vi "All time (SILAR).vi"(0 "Необходимое кол-во циклов":i32=1, 1 "Режим погружения подложки":u16(ring) items=["Частичное", "Полное"], 2 "Подъема подложки над раствором":dbl[](array[numeric])=[2.9, 2.9, 0.0, 0.0], 3 "Подъема подложки из раствора":dbl[](array[numeric])=[1.9, 1.9, 0.0, 0.0], 4 "Нахождения в растворе (секунды)":dbl[](array[numeric])=[1.0, 1.0, 0.0, 0.0] caption="Время нахождения в растворе (секунды)", 5 "Кол-во используемых растворов":i32(ring)=1 items=["Один"=1, "Два"=2, "Три"=3, "Четыре"=4], 6 "Высота стакана (мм)":dbl=50.0, 7 "Кол-во погружений в каждый стакан за один цикл":i32[](array[numeric])=[1, 1, 0, 0], 8 "Задержка после подъема из раствора (секунды)":dbl[](array[numeric])=[1.0, 1.0, 0.0, 0.0], 9 "Опускания подложки в раствор":dbl[](array[numeric])=[1.9, 1.9, 0.0, 0.0], 11 "Глубина погружения в раствор (мм)":dbl[](array[numeric])=[7.0, 7.0, 0.0, 0.0], 12 "Опускания подложки до раствора":dbl[](array[numeric])=[2.9, 2.9, 0.0, 0.0], 13 "Высота подложки (мм)":dbl=10.0, 14 "Кол-во жидкости в каждом стакане (мм)":dbl[](array[numeric])=[25.0, 25.0, 25.0, 25.0]) -> (10 "Все время":timestamp=timestamp(-14394 s since 1904-01-01) format="%<%H:%M:%S>T", 15 "Все время":dbl=6.0)   [LabVIEW 2016]
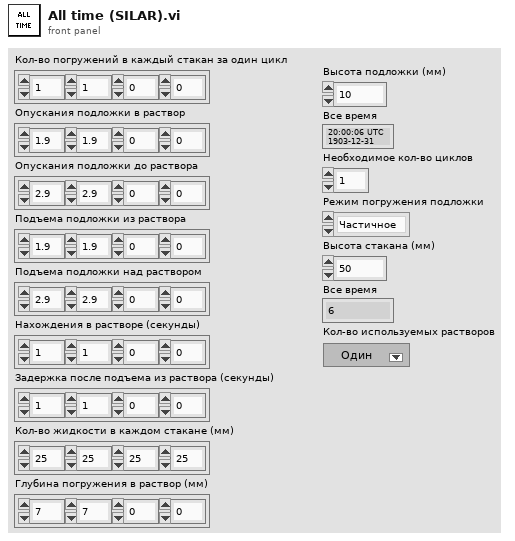
[diagram p1: front panel]
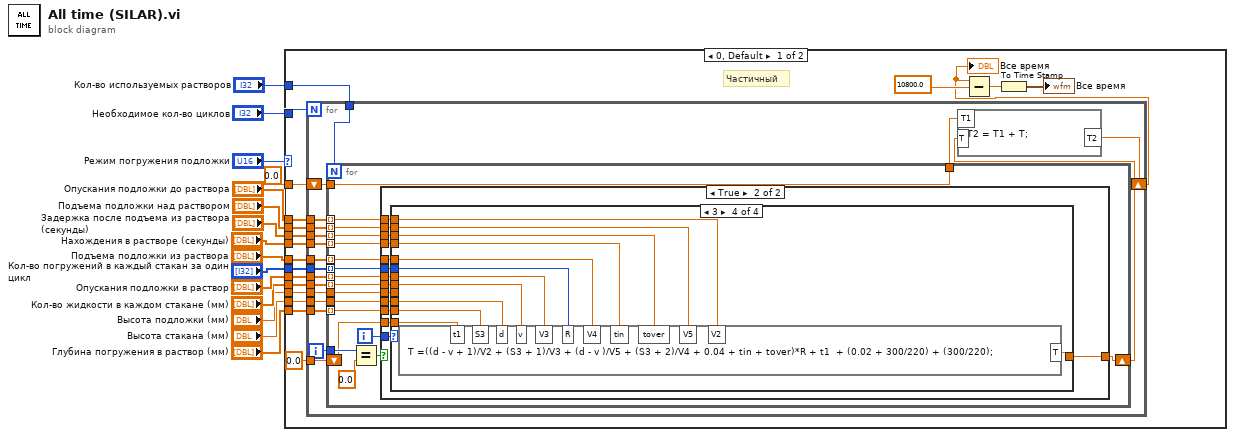
[diagram p0: block diagram]
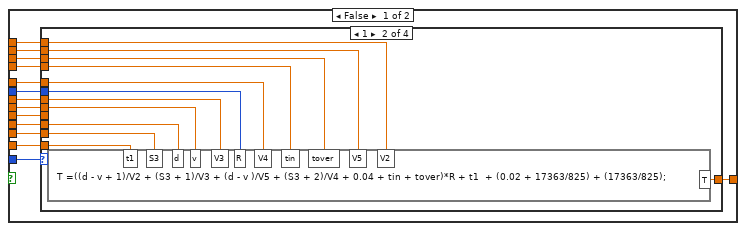
[diagram p2: hidden frame]
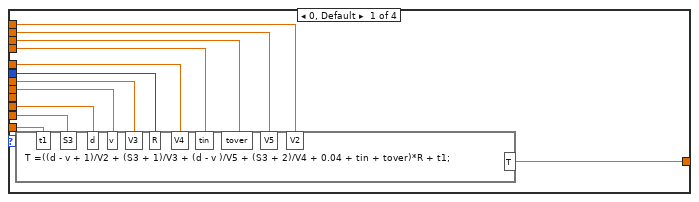
[diagram p3: hidden frame]
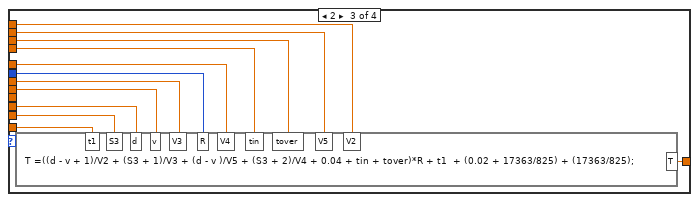
[diagram p4: hidden frame]
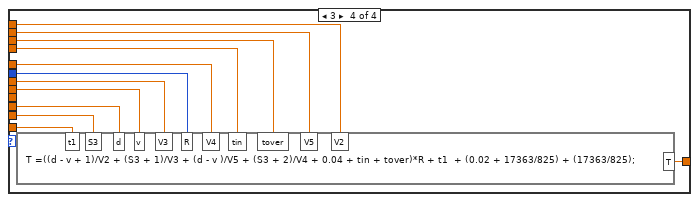
[diagram p5: hidden frame]
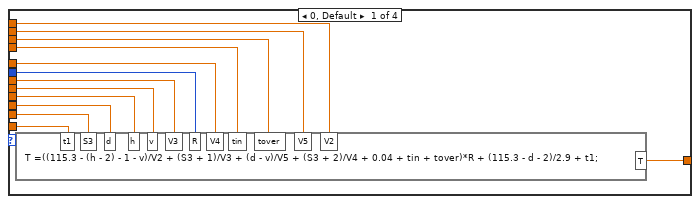
[diagram p6: hidden frame]
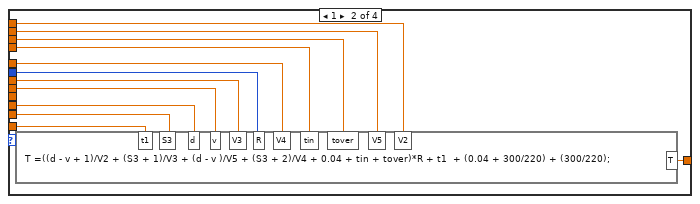
[diagram p7: hidden frame]
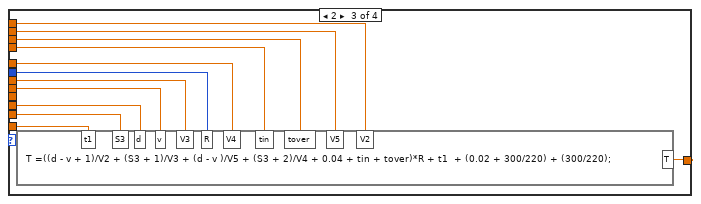
[diagram p8: hidden frame]
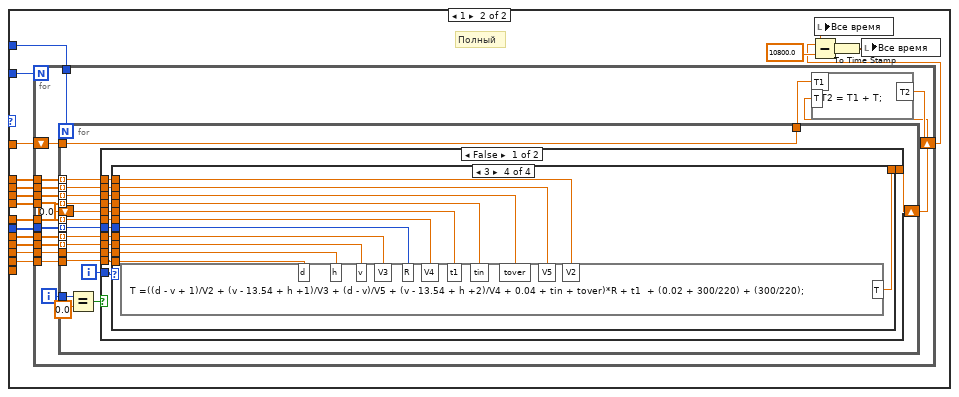
[diagram p9: hidden frame]
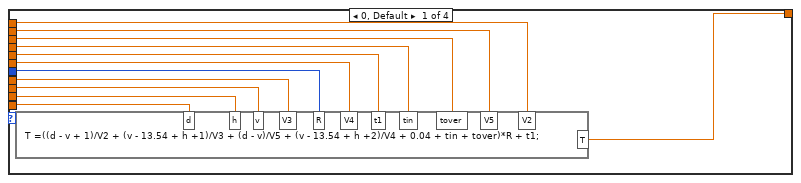
[diagram p10: hidden frame]
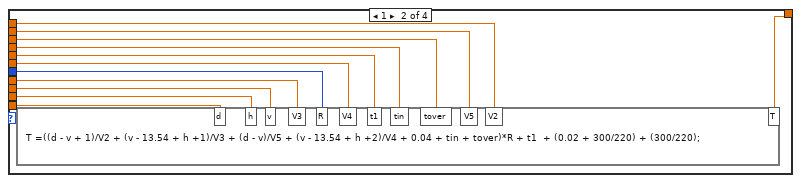
[diagram p11: hidden frame]
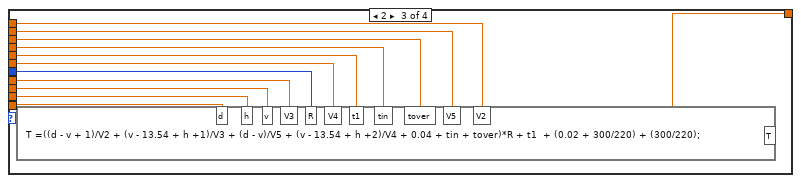
[diagram p12: hidden frame]
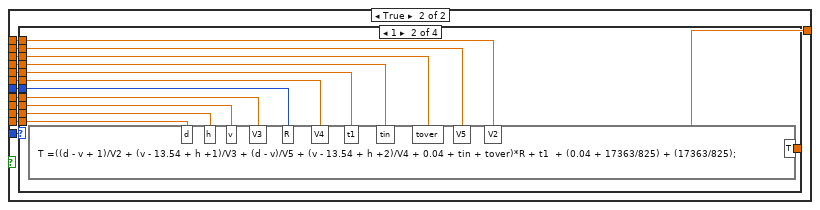
[diagram p13: hidden frame]
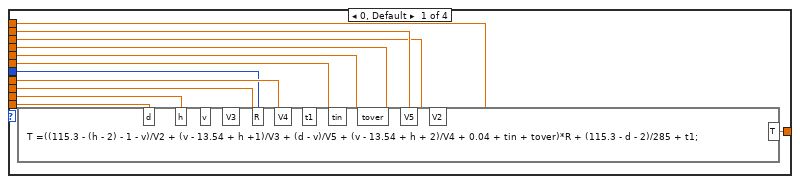
[diagram p14: hidden frame]
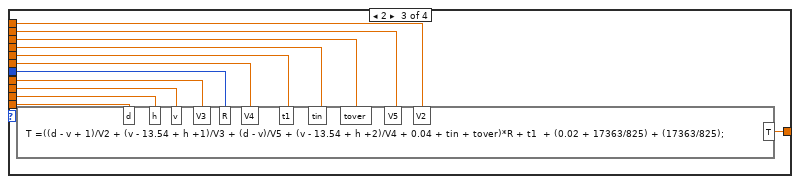
[diagram p15: hidden frame]
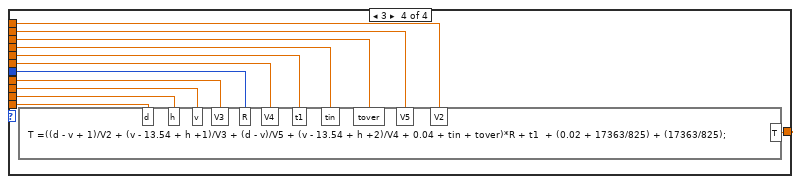
[diagram p16: hidden frame]
diagram:
  n1 = case shown="0, Default" "Режим погружения подложки" {
    tunnel: "Кол-во используемых растворов" -> [w33 w210]
    tunnel: "Задержка после подъема из раствора (секунды)" -> [w30 w206]
    tunnel: "Нахождения в растворе (секунды)" -> [w29 w205]
    tunnel: "Подъема подложки из раствора" -> [w28 w204]
    tunnel: "Кол-во погружений в каждый стакан за один цикл" -> [w22 w203]
    tunnel: "Опускания подложки в раствор" -> [w27 w202]
    tunnel: "Необходимое кол-во циклов" -> [w34 w209]
    tunnel: "Глубина погружения в раствор (мм)" -> [w26 _]
    tunnel: "Кол-во жидкости в каждом стакане (мм)" -> [w25 w201]
    tunnel: "Высота подложки (мм)" -> [w24 w200]
    tunnel: "Высота стакана (мм)" -> [w23 w199]
    tunnel: "Опускания подложки до раствора" -> [w32 w208]
    tunnel: "Подъема подложки над раствором" -> [w31 w207]
    tunnel: 0.0 -> [w18 w197]
    frame 0, Default {
      # "Частичный"
      n2 = for {
        N: w34 -> [_]
        tunnel: w33 -> [w52]
        shift-right: [w37] -> w16
        shift-left: w18 -> [w39]
        tunnel: w32 -> [w50]
        tunnel: w31 -> [w49]
        tunnel: w30 -> [w48]
        tunnel: w29 -> [w47]
        tunnel: w28 -> [w46]
        tunnel: w27 -> [w45]
        tunnel: w26 -> [w44]
        tunnel: w25 -> [w43]
        tunnel: w24 -> [w42]
        tunnel: w23 -> [w41]
        tunnel: w22 -> [w40]
        tunnel: 0.0 -> [w36]
        i -> [w51]
        n3 = for {
          N: w52 -> [_]
          shift-right: [w65] -> w35
          shift-left: w36 -> [w66]
          tunnel: w51 -> [w69]
          tunnel: w50 -> [w64] mode=indexing
          tunnel: w49 -> [w63] mode=indexing
          tunnel: w48 -> [w62] mode=indexing
          tunnel: w47 -> [w61] mode=indexing
          tunnel: w46 -> [w60] mode=indexing
          tunnel: w45 -> [w59] mode=indexing
          tunnel: w44 -> [w58] mode=indexing
          tunnel: w43 -> [w57] mode=indexing
          tunnel: w42 -> [w56]
          tunnel: w41 -> [w55]
          tunnel: w40 -> [w54] mode=indexing
          tunnel: w39 -> [w53]
          tunnel: [w53] -> w38
          i -> [w67]
          n4 = Equal?(x=w69, y=0.0) -> (x = y?=w68:bool)
          n5 = case shown="True" w68 {
            tunnel: w67 -> [w71 w146]
            tunnel: w66 -> [w79 w145]
            tunnel: [w84 w144] -> w65
            tunnel: w64 -> [w83 w143]
            tunnel: w63 -> [w82 w142]
            tunnel: w62 -> [w81 w141]
            tunnel: w61 -> [w80 w140]
            tunnel: w60 -> [w78 w139]
            tunnel: w59 -> [w76 w138]
            tunnel: w58 -> [w75 w137]
            tunnel: w57 -> [w74 w136]
            tunnel: w56 -> [w73 w135]
            tunnel: w55 -> [w72 w134]
            tunnel: w54 -> [w77 w133]
            frame False {
              n6 = case shown="1" w71 {
                tunnel: w79 -> [w96 w108 w119 w128]
                tunnel: [w95 w97 w110 w122] -> w84
                tunnel: w83 -> [w94 w107 w115 w132]
                tunnel: w82 -> [w93 w106 w116 w131]
                tunnel: w81 -> [w92 w105 w117 w130]
                tunnel: w80 -> [w91 w104 w118 w129]
                tunnel: w78 -> [w90 w103 w120 w127]
                tunnel: w76 -> [w89 w102 w114 w126]
                tunnel: w75 -> [w88 w101 w113 w125]
                tunnel: w74 -> [w85 w100 w112 w124]
                tunnel: w73 -> [_ _ _ _]
                tunnel: w72 -> [w87 w99 w111 w123]
                tunnel: w77 -> [w86 w98 w109 w121]
                frame 0, Default {
                  n7 = formula code="T =((d - v + 1)/V2 + (S3 + 1)/V3 + (d - v )/V5 + (S3 + 2)/V4 + 0.04 + tin + tover)*R + t1;"("t1"=w96, "v"=w85, "V2"=w94, "S3"=w88, "V3"=w89, "d"=w87, "V5"=w93, "V4"=w90, "tin"=w91, "tover"=w92, "R"=w86) -> ("T"=w95:dbl)
                }
                frame 1 {
                  n8 = formula code="T =((d - v + 1)/V2 + (S3 + 1)/V3 + (d - v )/V5 + (S3 + 2)/V4 + 0.04 + tin + tover)*R + t1  + (0.02 + 17363/825) + (17363/825);"("t1"=w108, "v"=w100, "V2"=w107, "S3"=w101, "V3"=w102, "d"=w99, "V5"=w106, "V4"=w103, "tin"=w104, "tover"=w105, "R"=w98) -> ("T"=w97:dbl)
                }
                frame 2 {
                  n9 = formula code="T =((d - v + 1)/V2 + (S3 + 1)/V3 + (d - v )/V5 + (S3 + 2)/V4 + 0.04 + tin + tover)*R + t1  + (0.02 + 17363/825) + (17363/825);"("t1"=w119, "v"=w112, "V2"=w115, "S3"=w113, "V3"=w114, "d"=w111, "V5"=w116, "V4"=w120, "tin"=w118, "tover"=w117, "R"=w109) -> ("T"=w110:dbl)
                }
                frame 3 {
                  n10 = formula code="T =((d - v + 1)/V2 + (S3 + 1)/V3 + (d - v )/V5 + (S3 + 2)/V4 + 0.04 + tin + tover)*R + t1  + (0.02 + 17363/825) + (17363/825);"("t1"=w128, "v"=w124, "V2"=w132, "S3"=w125, "V3"=w126, "d"=w123, "V5"=w131, "V4"=w127, "tin"=w129, "tover"=w130, "R"=w121) -> ("T"=w122:dbl)
                }
              }
            }
            frame True {
              n11 = case shown="3" w146 {
                tunnel: w145 -> [w159 w171 w172 w191]
                tunnel: [w158 w160 w174 w186] -> w144
                tunnel: w143 -> [w157 w170 w179 w195]
                tunnel: w142 -> [w156 w169 w180 w194]
                tunnel: w141 -> [w155 w168 w181 w193]
                tunnel: w140 -> [w154 w167 w182 w192]
                tunnel: w139 -> [w153 w166 w183 w190]
                tunnel: w138 -> [w152 w165 w178 w189]
                tunnel: w137 -> [w151 w164 w177 w184]
                tunnel: w136 -> [w150 w163 w176 w188]
                tunnel: w135 -> [w149 _ _ _]
                tunnel: w134 -> [w148 w162 w175 w187]
                tunnel: w133 -> [w147 w161 w173 w185]
                frame 0, Default {
                  n12 = formula code="T =((115.3 - (h - 2) - 1 - v)/V2 + (S3 + 1)/V3 + (d - v)/V5 + (S3 + 2)/V4 + 0.04 + tin + tover)*R + (115.3 - d - 2)/2.9 + t1;"("t1"=w159, "v"=w150, "h"=w149, "V2"=w157, "S3"=w151, "V3"=w152, "d"=w148, "V5"=w156, "V4"=w153, "tin"=w154, "tover"=w155, "R"=w147) -> ("T"=w158:dbl)
                }
                frame 1 {
                  n13 = formula code="T =((d - v + 1)/V2 + (S3 + 1)/V3 + (d - v )/V5 + (S3 + 2)/V4 + 0.04 + tin + tover)*R + t1  + (0.04 + 300/220) + (300/220);"("t1"=w171, "v"=w163, "V2"=w170, "S3"=w164, "V3"=w165, "d"=w162, "V5"=w169, "V4"=w166, "tin"=w167, "tover"=w168, "R"=w161) -> ("T"=w160:dbl)
                }
                frame 2 {
                  n14 = formula code="T =((d - v + 1)/V2 + (S3 + 1)/V3 + (d - v )/V5 + (S3 + 2)/V4 + 0.04 + tin + tover)*R + t1  + (0.02 + 300/220) + (300/220);"("t1"=w172, "v"=w176, "V2"=w179, "S3"=w177, "V3"=w178, "d"=w175, "V5"=w180, "V4"=w183, "tin"=w182, "tover"=w181, "R"=w173) -> ("T"=w174:dbl)
                }
                frame 3 {
                  n15 = formula code="T =((d - v + 1)/V2 + (S3 + 1)/V3 + (d - v )/V5 + (S3 + 2)/V4 + 0.04 + tin + tover)*R + t1  + (0.02 + 300/220) + (300/220);"("t1"=w191, "v"=w188, "V2"=w195, "S3"=w184, "V3"=w189, "d"=w187, "V5"=w194, "V4"=w190, "tin"=w192, "tover"=w193, "R"=w185) -> ("T"=w186:dbl)
                }
              }
            }
          }
        }
        n16 = formula code="T2 = T1 + T;"("T1"=w38, "T"=w35) -> ("T2"=w37:dbl)
      }
      "Все время" <- w16
      n17 = Subtract(x=w16, y=10800.0) -> (x-y=w20:dbl)
      n18 = To Time Stamp(1:w20) -> (0:→"Все время":timestamp)
    }
    frame 1 {
      # "Полный"
      n19 = for {
        N: w209 -> [_]
        tunnel: w210 -> [w229]
        shift-right: [w215] -> w196
        shift-left: w197 -> [w217]
        tunnel: w208 -> [w226]
        tunnel: w207 -> [w225]
        tunnel: w206 -> [w224]
        tunnel: w205 -> [w223]
        tunnel: w204 -> [w222]
        tunnel: w202 -> [w221]
        tunnel: w201 -> [w220]
        tunnel: w200 -> [w213]
        tunnel: w199 -> [w219]
        tunnel: w203 -> [w218]
        i -> [w228]
        n20 = for {
          N: w229 -> [_]
          shift-right: [w241] -> w214
          shift-left: 0.0 -> [w242]
          tunnel: w228 -> [w245]
          tunnel: w226 -> [w240] mode=indexing
          tunnel: w225 -> [w239] mode=indexing
          tunnel: w224 -> [w238] mode=indexing
          tunnel: w223 -> [w237] mode=indexing
          tunnel: w222 -> [w236] mode=indexing
          tunnel: w221 -> [w235] mode=indexing
          tunnel: w220 -> [w234] mode=indexing
          tunnel: w219 -> [w233]
          tunnel: w218 -> [w232] mode=indexing
          tunnel: w217 -> [w231]
          tunnel: [w231] -> w216
          tunnel: w213 -> [w230]
          i -> [w243]
          n21 = Equal?(x=w245, y=0.0) -> (x = y?=w244:bool)
          n22 = case shown="False" w244 {
            tunnel: w243 -> [w249 w320]
            tunnel: w242 -> [w255 w319]
            tunnel: [w247 w318] -> w241
            tunnel: w240 -> [w259 w317]
            tunnel: w239 -> [w258 w316]
            tunnel: w238 -> [w257 w315]
            tunnel: w237 -> [w256 w314]
            tunnel: w236 -> [w254 w313]
            tunnel: w235 -> [w252 w312]
            tunnel: w234 -> [w251 w311]
            tunnel: w233 -> [w250 w310]
            tunnel: w232 -> [w253 w309]
            tunnel: w230 -> [w248 w308]
            frame False {
              n23 = case shown="3" w249 {
                tunnel: w255 -> [w271 w283 w294 w303]
                tunnel: [w270 w273 w286 w298] -> w247
                tunnel: w259 -> [w269 w282 w290 w307]
                tunnel: w258 -> [w268 w281 w291 w306]
                tunnel: w257 -> [w267 w280 w292 w305]
                tunnel: w256 -> [w266 w279 w293 w304]
                tunnel: w254 -> [w265 w278 w295 w302]
                tunnel: w252 -> [w264 w277 w289 w301]
                tunnel: w251 -> [w263 w276 w288 w300]
                tunnel: w250 -> [w262 w275 w287 w299]
                tunnel: w253 -> [w261 w274 w285 w297]
                tunnel: w248 -> [w260 w272 w284 w296]
                frame 0, Default {
                  n24 = formula code="T =((d - v + 1)/V2 + (v - 13.54 + h +1)/V3 + (d - v)/V5 + (v - 13.54 + h +2)/V4 + 0.04 + tin + tover)*R + t1;"("t1"=w271, "v"=w263, "V2"=w269, "V3"=w264, "d"=w262, "V5"=w268, "V4"=w265, "tin"=w266, "tover"=w267, "R"=w261, "h"=w260) -> ("T"=w270:dbl)
                }
                frame 1 {
                  n25 = formula code="T =((d - v + 1)/V2 + (v - 13.54 + h +1)/V3 + (d - v)/V5 + (v - 13.54 + h +2)/V4 + 0.04 + tin + tover)*R + t1  + (0.02 + 300/220) + (300/220);"("t1"=w283, "v"=w276, "V2"=w282, "V3"=w277, "d"=w275, "V5"=w281, "V4"=w278, "tin"=w279, "tover"=w280, "R"=w274, "h"=w272) -> ("T"=w273:dbl)
                }
                frame 2 {
                  n26 = formula code="T =((d - v + 1)/V2 + (v - 13.54 + h +1)/V3 + (d - v)/V5 + (v - 13.54 + h +2)/V4 + 0.04 + tin + tover)*R + t1  + (0.02 + 300/220) + (300/220);"("t1"=w294, "v"=w288, "V2"=w290, "V3"=w289, "d"=w287, "V5"=w291, "V4"=w295, "tin"=w293, "tover"=w292, "R"=w285, "h"=w284) -> ("T"=w286:dbl)
                }
                frame 3 {
                  n27 = formula code="T =((d - v + 1)/V2 + (v - 13.54 + h +1)/V3 + (d - v)/V5 + (v - 13.54 + h +2)/V4 + 0.04 + tin + tover)*R + t1  + (0.02 + 300/220) + (300/220);"("t1"=w303, "v"=w300, "V2"=w307, "V3"=w301, "d"=w299, "V5"=w306, "V4"=w302, "tin"=w304, "tover"=w305, "R"=w297, "h"=w296) -> ("T"=w298:dbl)
                }
              }
            }
            frame True {
              n28 = case shown="1" w320 {
                tunnel: w319 -> [w332 w344 w355 w364]
                tunnel: [w331 w334 w347 w359] -> w318
                tunnel: w317 -> [w330 w343 w351 w368]
                tunnel: w316 -> [w329 w342 w352 w367]
                tunnel: w315 -> [w328 w341 w353 w366]
                tunnel: w314 -> [w327 w340 w354 w365]
                tunnel: w313 -> [w326 w339 w356 w363]
                tunnel: w312 -> [w325 w338 w350 w362]
                tunnel: w311 -> [w324 w337 w349 w361]
                tunnel: w310 -> [w323 w336 w348 w360]
                tunnel: w309 -> [w322 w335 w346 w358]
                tunnel: w308 -> [w321 w333 w345 w357]
                frame 0, Default {
                  n29 = formula code="T =((115.3 - (h - 2) - 1 - v)/V2 + (v - 13.54 + h +1)/V3 + (d - v)/V5 + (v - 13.54 + h + 2)/V4 + 0.04 + tin + tover)*R + (115.3 - d - 2)/285 + t1;"("t1"=w332, "v"=w324, "h"=w321, "V2"=w330, "V3"=w325, "d"=w323, "V5"=w329, "V4"=w326, "tin"=w327, "tover"=w328, "R"=w322) -> ("T"=w331:dbl)
                }
                frame 1 {
                  n30 = formula code="T =((d - v + 1)/V2 + (v - 13.54 + h +1)/V3 + (d - v)/V5 + (v - 13.54 + h +2)/V4 + 0.04 + tin + tover)*R + t1  + (0.04 + 17363/825) + (17363/825);"("t1"=w344, "v"=w337, "V2"=w343, "V3"=w338, "d"=w336, "V5"=w342, "V4"=w339, "tin"=w340, "tover"=w341, "R"=w335, "h"=w333) -> ("T"=w334:dbl)
                }
                frame 2 {
                  n31 = formula code="T =((d - v + 1)/V2 + (v - 13.54 + h +1)/V3 + (d - v)/V5 + (v - 13.54 + h +2)/V4 + 0.04 + tin + tover)*R + t1  + (0.02 + 17363/825) + (17363/825);"("t1"=w355, "v"=w349, "V2"=w351, "V3"=w350, "d"=w348, "V5"=w352, "V4"=w356, "tin"=w354, "tover"=w353, "R"=w346, "h"=w345) -> ("T"=w347:dbl)
                }
                frame 3 {
                  n32 = formula code="T =((d - v + 1)/V2 + (v - 13.54 + h +1)/V3 + (d - v)/V5 + (v - 13.54 + h +2)/V4 + 0.04 + tin + tover)*R + t1  + (0.02 + 17363/825) + (17363/825);"("t1"=w364, "v"=w361, "V2"=w368, "V3"=w362, "d"=w360, "V5"=w367, "V4"=w363, "tin"=w365, "tover"=w366, "R"=w358, "h"=w357) -> ("T"=w359:dbl)
                }
              }
            }
          }
        }
        n33 = formula code="T2 = T1 + T;"("T1"=w216, "T"=w214) -> ("T2"=w215:dbl)
      }
      n34 = Subtract(x=w196, y=10800.0) -> (x-y=w211:dbl)
      n35 = local write "Все время"(w196) -> ()
      n36 = To Time Stamp(1:w211) -> (0:w198:timestamp)
      n37 = local write "Все время"(w198) -> ()
    }
  }
